vi "Translator.File.Read.Font.vi"(6 "Do not save font? (F)":bool, 8 "error in":errorcluster, 10 "Translation file in":path=path "D:/PL_0125_Sapphire_Automation_branches/SOFTWARE_v1.1-Translation/settings/Translation-Chinese.ini") -> (0 "error out":errorcluster, 1 "font name":string="abcdefghijklmnopqrstuvwxyz", 2 "Translation file out":path=path "D:/PL_0125_Sapphire_Automation_branches/SOFTWARE_v1.1-Translation/settings/Translation-Chinese.ini", 4 "restart required?":bool)   [LabVIEW 2019, in "Tools.lvlib"]
uses:
  Tools.lvlib
  Translator.Global.vi
  <vilib>/Utility/config.llb/Read Key (String).vi
  <vilib>/Utility/config.llb/Write Key (String).vi
  <vilib>/Utility/config.llb/NI_LVConfig.lvlib
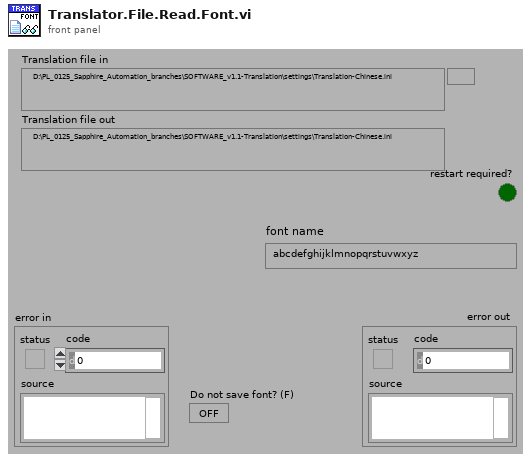
[diagram p1: front panel]
types:
  T1 = typedef "NI_LVConfig.lvlib/Config Data RefNum.ctl" = refnum<k1>
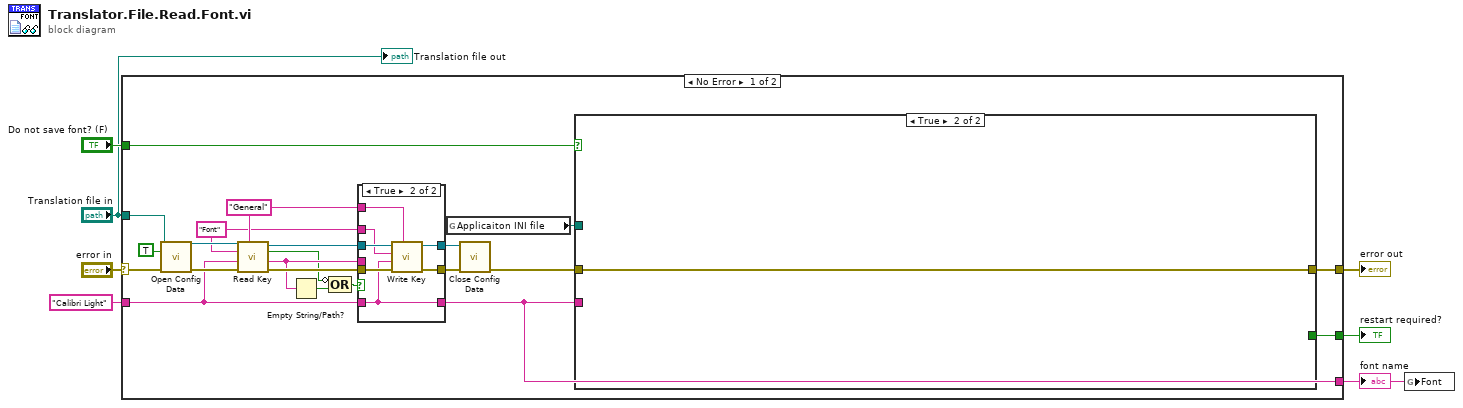
[diagram p0: block diagram]
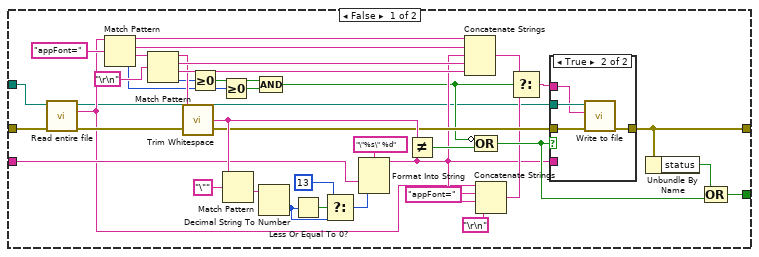
[diagram p2: hidden frame]
diagram:
  n1 = case shown="No Error" "error in" {
    selector: "error in" -> [w18 w84]
    tunnel: [w13 w84] -> w7
    tunnel: "Translation file in" -> [w19 _]
    tunnel: [w11 w83] -> w4
    tunnel: "Calibri Light" ("default value") -> [w20 w83]
    tunnel: [w12 _] -> w3
    tunnel: "Do not save font? (F)" -> [w10 _]
    frame No Error {
      w21 = "Font" ("section")
      w22 = "General" ("section")
      n2 = call <vilib>:"Open Config Data.vi"("error in (no error)"=w18, "create file if necessary (T)"=TRUE, "configuration file path"=w19) -> ("error out"=w28:errorcluster, "refnum"=w27:T1)  [unwired: 6 in, 1 out]
      n3 = call-poly <vilib>:"Read Key.vi"("section"=w22, "error in (no error)"=w28, "default value"=w20, "key"=w21, "refnum"=w27) -> ("error out"=w26:errorcluster, "value"=w17:string, "found?"=w15:bool, "refnum out"=w23:T1)  [unwired: 3 in]
      n4 = Empty String/Path?(string/path=w17) -> (empty?=w16:bool)
      n5 = Compound Arithmetic op=OR(invert w15, w16) -> (w14:bool)
      n6 = case shown="True" w14 {
        tunnel: w26 -> [w75 w82]
        tunnel: [w75 w81] -> w25
        tunnel: [w74 w80] -> w24
        tunnel: w23 -> [w74 w79]
        tunnel: w22 -> [_ w78]
        tunnel: w21 -> [_ w77]
        tunnel: w17 -> [w73 _]
        tunnel: w20 -> [_ w76]
        tunnel: [w73 w76] -> w11
        frame False {
        }
        frame True {
          n7 = call-poly <vilib>:"Write Key.vi"("section"=w78, "error in (no error)"=w82, "value"=w76, "key"=w77, "refnum"=w79) -> ("error out"=w81:errorcluster, "refnum out"=w80:T1)  [unwired: 4 in, 1 out]
        }
      }
      n8 = global read "Translator.Global.vi" "Applicaiton INI file"() -> (w9:path)
      n9 = call <vilib>:"Close Config Data.vi"("error in (no error)"=w25, "refnum"=w24) -> ("error out"=w8:errorcluster)  [unwired: 8 in, 1 out]
      n10 = case shown="True" w10 {
        tunnel: w8 -> [w30 w72]
        tunnel: w11 -> [w47 _]
        tunnel: [w34 w72] -> w13
        tunnel: [w33 _] -> w12
        tunnel: w9 -> [w31 _]
        frame False {
          n11 = call "Read entire file.vi"("error in"=w30, "file"=w31) -> ("error out"=w54:errorcluster, "contents"=w41:string)  [unwired: 4 in]
          n12 = Match Pattern(string=w41, regular expression="appFont=" ("section")) -> (before substring=w52:string, match substring=w53:string, after substring=w49:string, offset past match=w39:i32)  [unwired: 1 in]
          n13 = Match Pattern(string=w49, regular expression="\r\n") -> (before substring=w48:string, match substring=w51:string, after substring=w50:string, offset past match=w40:i32)  [unwired: 1 in]
          n14 = call <vilib>:"Trim Whitespace.vi"("string"=w48) -> ("trimmed string"=w55:string)  [unwired: 1 in]
          n15 = Greater Or Equal To 0?(x=w40) -> (x >= 0?=w38:bool)
          n16 = Greater Or Equal To 0?(x=w39) -> (x >= 0?=w37:bool)
          n17 = Match Pattern(string=w55, regular expression="\"") -> (after substring=w56:string)  [unwired: 1 in, 3 out]
          n18 = Decimal String To Number(string=w56) -> (number=w61:i32)  [unwired: 2 in, 1 out]
          n19 = Compound Arithmetic op=AND(w38, w37) -> (w36:bool)
          n20 = Less Or Equal To 0?(x=w61) -> (x <= 0?=w62:bool)
          n21 = Select(t=13, s=w62, f=w61) -> (s? t:f=w60:i32)
          n22 = Format Into String(format string="\"%s\" %d", w47, w60) -> (resulting string=w43:string)  [unwired: 2 in, 1 out]
          n23 = Not Equal?(x=w55, y=w43) -> (x != y?=w66:bool)
          n24 = Concatenate Strings(w52, w53, w43, w51, w50) -> (w35:string)
          n25 = Compound Arithmetic op=OR(invert w36, w66) -> (w65:bool)
          n26 = Concatenate Strings(w41, "appFont=" ("string"), w43, "\r\n") -> (w44:string)
          n27 = Select(t=w35, s=w36, f=w44) -> (s? t:f=w42:string)
          n28 = case shown="True" w65 {
            tunnel: w54 -> [w67 w71]
            tunnel: [w67 w70] -> w34
            tunnel: w43 -> [_ _]
            tunnel: w31 -> [_ w69]
            tunnel: w42 -> [_ w68]
            frame False {
            }
            frame True {
              n29 = call "Write to file.vi"("error in"=w71, "addition"=w68, "file"=w69) -> ("error out"=w70:errorcluster)  [unwired: 8 in]
            }
          }
          n30 = Unbundle By Name(w34) -> ("status"=w32:bool)
          n31 = Compound Arithmetic op=OR(w32, w65) -> (w33:bool)
        }
        frame True {
        }
      }
    }
    frame Error {
    }
  }
  "error out" <- w7
  "font name" <- w4
  "restart required?" <- w3
  n32 = global write "Translator.Global.vi" "Font"(w4) -> ()
  "Translation file out" <- "Translation file in"
